vi "TestEthConnection x2.vi"(8 "IP address 2":string="172.16.14.23", 9 "ENA2":bool caption="Connection 2 enable", 10 "IP address 1":string="172.16.14.22", 11 "ENA1":bool caption="Connection 1 enable") -> (0 "error out":errorcluster, 1 "Answers OK?":bool)   [LabVIEW 2015, in "VIPM2.lvlib"]
doc: "Testeja 2 Eth connections amb reentrança."
uses:
  VIPM2.lvlib
panel:
  out "Answer to open 1":string="\n\r\n"
  out "Answer to open 2":string="\n\r\n"
  # "Test Ethernet Connections"
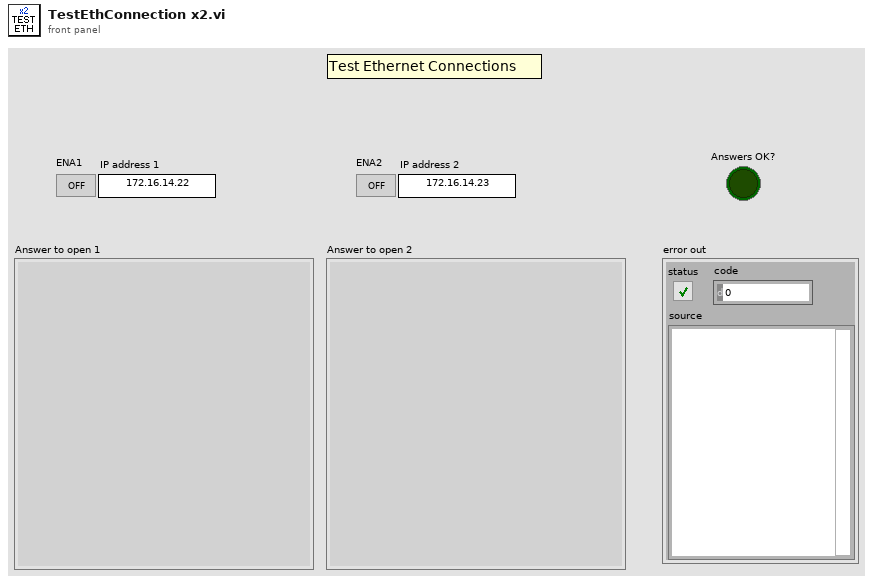
[diagram p1: front panel]
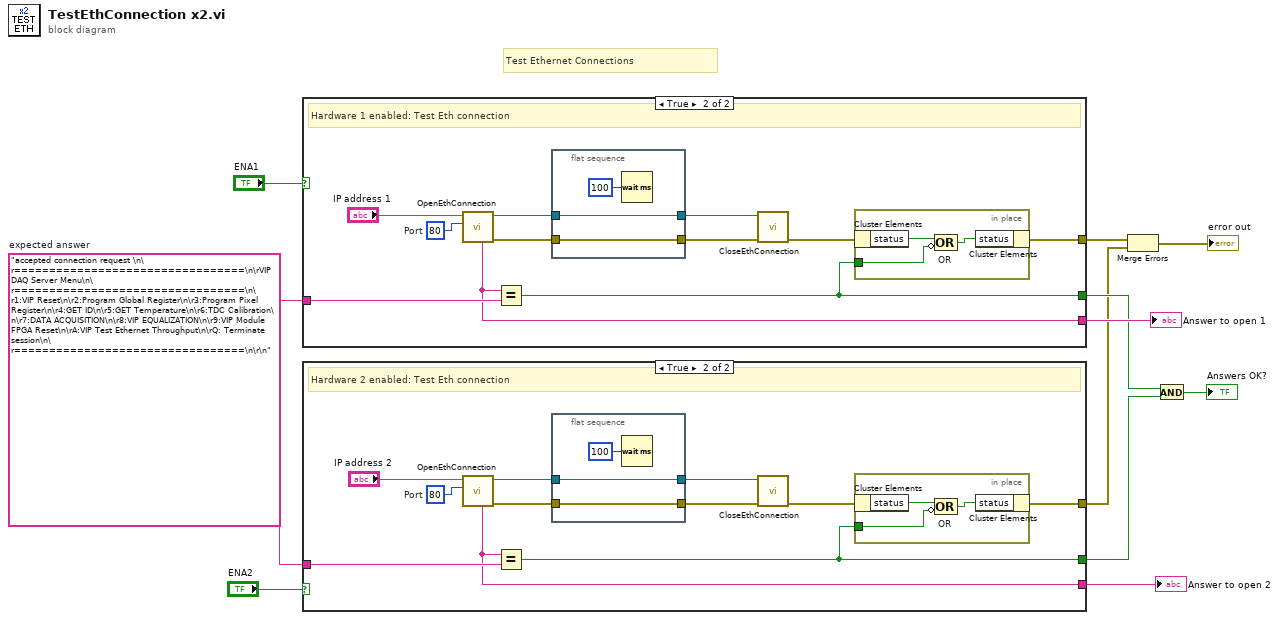
[diagram p0: block diagram]
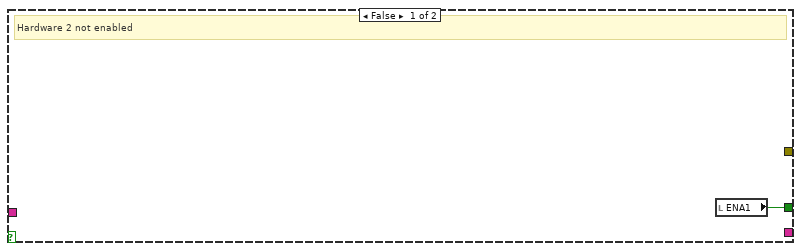
[diagram p2: hidden frame]
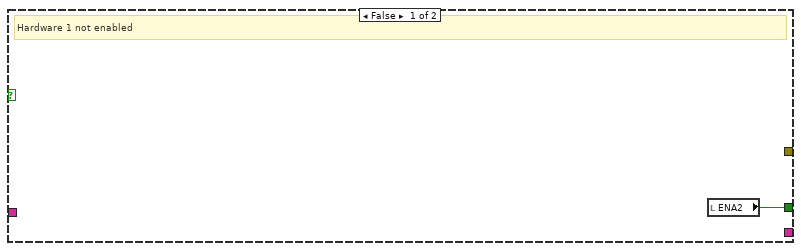
[diagram p3: hidden frame]
diagram:
  w9 = "accepted connection request \n\r=================================\n\rVIP DAQ Server Menu\n\r=================================\n\r1:VIP Reset\n\r2:Program Global Register\n\r3:Program Pixel Register\n\r4:GET ID\n\r5:GET Temperature\n\r6:TDC Calibration\n\r7:DATA ACQUISITION\n\r8:VIP EQUALIZATION\n\r9:VIP Module FPGA Reset\n\rA:VIP Test Ethernet Throughput\n\rQ: Terminate session\n\r=================================\n\r\n"  # expected answer
  # "Test Ethernet Connections"
  n1 = case shown="True" "ENA1" {
    tunnel: w9 -> [_ w23]
    tunnel: [w12 w16] -> w6
    tunnel: [_ w15] -> w11
    tunnel: [_ w13] -> w3
    frame False {
      # "Hardware 1 not enabled"
      n2 = local read "ENA2"() -> (w12:bool)
    }
    frame True {
      w18 = u16 80  # Port
      # "Hardware 1 enabled: Test Eth connection"
      n3 = call "OpenEthConnection.vi"("Port"=w18, "IP address"="IP address 1") -> ("error out"=w22:errorcluster, "connection ID out"=w19:refnum<k5>, "Answer"=w15:string)  [unwired: 7 in]
      n4 = Equal?(x=w15, y=w23) -> (x = y?=w16:bool)
      n5 = flat-sequence {
        tunnel: w22 -> [w29]
        tunnel: [w29] -> w21
        tunnel: [w28] -> w20
        tunnel: w19 -> [w28]
        frame #0 {
          n6 = Wait (ms)(milliseconds to wait=u32 100) -> ()  [unwired: 1 out]
        }
      }
      n7 = call "CloseEthConnection.vi"("error in (no error)"=w21, "connection ID"=w20) -> ("error out"=w17:errorcluster)  [unwired: 9 in]
      n8 = in-place "In Place Element Structure" {
        in-place-border: w16 -> [w24]
        n9 = in-place-cluster #1(w17) -> ("status"=w26:bool)
        n10 = Compound Arithmetic op=OR "OR"(w26, invert w24) -> (w25:bool)
        n11 = in-place-cluster #1("status"=w25) -> (w13:errorcluster)
      }
    }
  }
  "Answer to open 1" <- w11
  n12 = case shown="True" "ENA2" {
    tunnel: w9 -> [_ w41]
    tunnel: [w30 w34] -> w5
    tunnel: [_ w33] -> w7
    tunnel: [_ w31] -> w2
    frame False {
      # "Hardware 2 not enabled"
      n13 = local read "ENA1"() -> (w30:bool)
    }
    frame True {
      w36 = u16 80  # Port
      # "Hardware 2 enabled: Test Eth connection"
      n14 = call "OpenEthConnection.vi"("Port"=w36, "IP address"="IP address 2") -> ("error out"=w40:errorcluster, "connection ID out"=w37:refnum<k5>, "Answer"=w33:string)  [unwired: 7 in]
      n15 = Equal?(x=w33, y=w41) -> (x = y?=w34:bool)
      n16 = flat-sequence {
        tunnel: w40 -> [w47]
        tunnel: [w47] -> w39
        tunnel: [w46] -> w38
        tunnel: w37 -> [w46]
        frame #0 {
          n17 = Wait (ms)(milliseconds to wait=u32 100) -> ()  [unwired: 1 out]
        }
      }
      n18 = call "CloseEthConnection.vi"("error in (no error)"=w39, "connection ID"=w38) -> ("error out"=w35:errorcluster)  [unwired: 9 in]
      n19 = in-place "In Place Element Structure" {
        in-place-border: w34 -> [w42]
        n20 = in-place-cluster #2(w35) -> ("status"=w44:bool)
        n21 = Compound Arithmetic op=OR "OR"(w44, invert w42) -> (w43:bool)
        n22 = in-place-cluster #2("status"=w43) -> (w31:errorcluster)
      }
    }
  }
  "Answer to open 2" <- w7
  n23 = Merge Errors "Merge Errors"(w3, w2) -> (→"error out":errorcluster)
  n24 = And(x=w6, y=w5) -> (x .and. y?=→"Answers OK?":bool)
